vi "Read Roughness.vi"(8 "error in (no error)":errorcluster, 11 "Video Cam Processor in":refnum<class "Video Cam Processor.lvclass">) -> (0 "error out":errorcluster, 3 "Video Cam Processor out":refnum<class "Video Cam Processor.lvclass">)   [LabVIEW 2018, in "Video Cam Processor.lvclass"]
uses:
  Video Cam Processor.lvclass
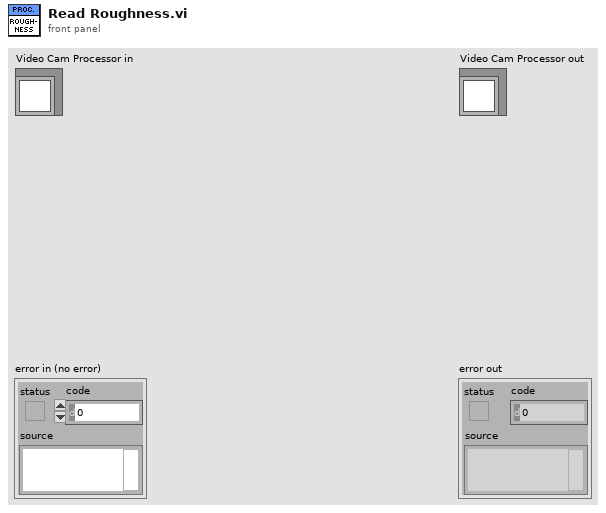
[diagram p1: front panel]
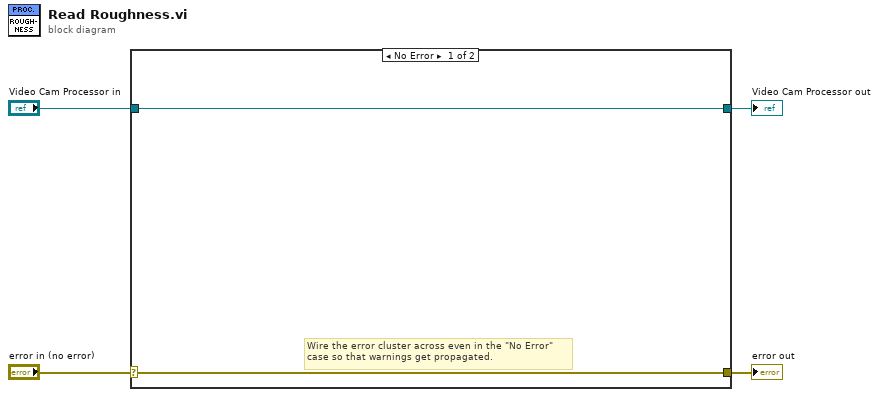
[diagram p0: block diagram]
diagram:
  n1 = case shown="No Error" "error in (no error)" {
    selector: "error in (no error)" -> [w5 w8]
    tunnel: [w5 w8] -> w3
    tunnel: [w6 w7] -> w1
    tunnel: "Video Cam Processor in" -> [w6 w7]
    frame No Error {
      # "Wire the error cluster across even in the \"No Error\"\ncase so that warnings get propagated."
    }
    frame Error {
    }
  }
  "error out" <- w3
  "Video Cam Processor out" <- w1
